vi "fetchChannelList.vi"(8 "error in":errorcluster, 10 "DAQ ID #":i32, 11 "Channels":string) -> (0 "error out":errorcluster, 2 "Channel Match?":bool, 3 "Read Channels":string)   [LabVIEW 2024]
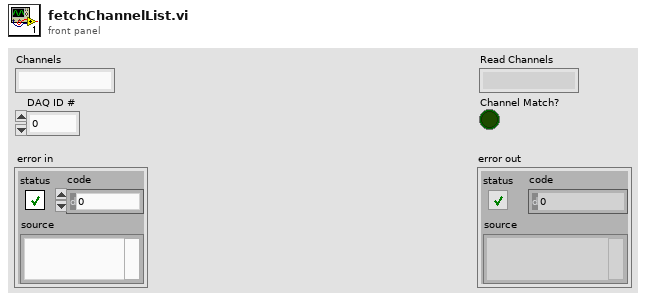
[diagram p1: front panel]
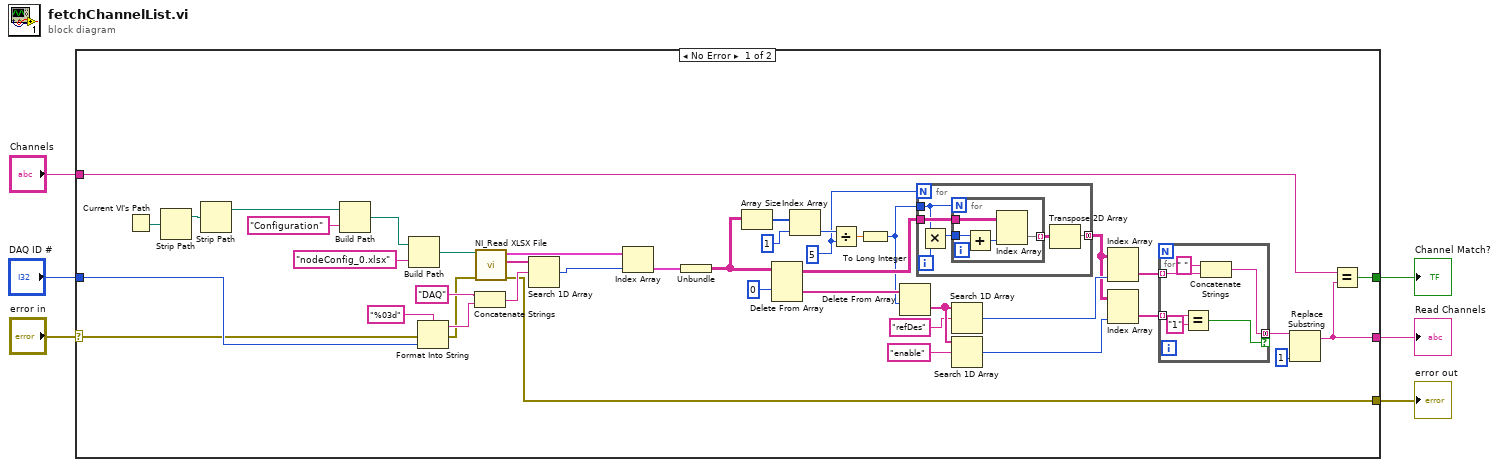
[diagram p0: block diagram]
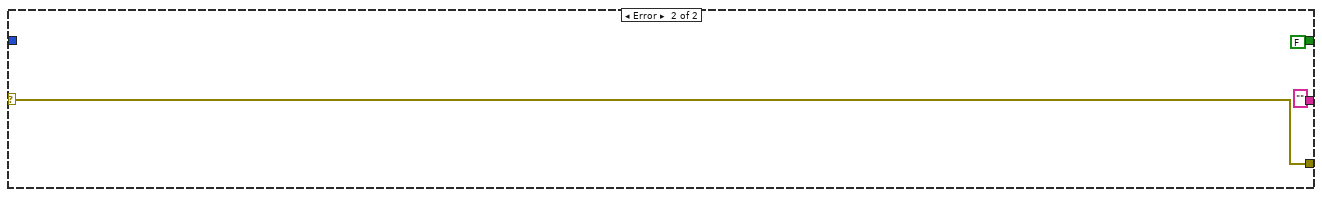
[diagram p2: hidden frame]
diagram:
  n1 = case shown="No Error" "error in" {
    selector: "error in" -> [w25 w66]
    tunnel: "DAQ ID #" -> [w32 _]
    tunnel: [w7 ""] -> w5
    tunnel: "Channels" -> [w15 _]
    tunnel: [w26 FALSE] -> w3
    tunnel: [w24 w66] -> w1
    frame No Error {
      w17 = 5 ("y")
      n2 = Current VI's Path() -> (path=w46:path)
      n3 = Strip Path(path=w46) -> (stripped path=w43:path)  [unwired: 1 out]
      n4 = Strip Path(path=w43) -> (stripped path=w42:path)  [unwired: 1 out]
      n5 = Build Path(base path=w42, name or relative path="Configuration") -> (appended path=w44:path)
      n6 = Build Path(base path=w44, name or relative path="nodeConfig_0.xlsx") -> (appended path=w47:path)
      n7 = Format Into String(format string="%03d", error in=w25, w32) -> (resulting string=w36:string, error out=w34:errorcluster)  [unwired: 1 in]
      n8 = Concatenate Strings("DAQ" ("string"), w36) -> (w38:string)
      n9 = call "NI_Read XLSX File.vi"("error in"=w34, "XLSX File"=w47) -> ("error out"=w24:errorcluster, "Sheet Names"=w39:string[], "Sheet Data"=w41:cluster{"Array":string[][]}[])  [unwired: 7 in]
      n10 = Search 1D Array(1D array=w39, element=w38) -> (index of element=w33:i32)  [unwired: 1 in]
      n11 = Index Array(array=w41, index=w33) -> (element=w40:cluster{"Array":string[][]})
      n12 = Unbundle(w40) -> ("Array"=w23:string[][])
      n13 = Array Size(array=w23) -> (size(s)=w31:i32[])
      n14 = Delete From Array(array=w23, index (row)=0) -> (deleted portion=w19:string[], array with subset deleted=w18:string[][])  [unwired: 2 in]
      n15 = Index Array(array=w31, index=1) -> (element=w29:i32)
      n16 = Divide(x=w29, y=w17) -> (x/y=w27:dbl)
      n17 = To Long Integer(number=w27) -> (32bit integer=w16:i32)
      n18 = Delete From Array(array=w19, length=w16) -> (deleted portion=w22:string[])  [unwired: 1 in, 1 out]
      n19 = for {
        N: w17 -> [_]
        tunnel: w18 -> [w60]
        tunnel: w16 -> [w58]
        tunnel: [w55] -> w13 mode=concatenating
        i -> [w59]
        n20 = Multiply(x=w58, y=w59) -> (x*y=w57:i32)
        n21 = for {
          N: w58 -> [_]
          tunnel: w60 -> [w65]
          tunnel: w57 -> [w63]
          tunnel: [w61] -> w56 mode=indexing
          i -> [w64]
          n22 = Add(x=w63, y=w64) -> (x+y=w62:i32)
          n23 = Index Array(array=w65, index (col)=w62) -> (element=w61:string[])  [unwired: 1 in]
        }
        n24 = Transpose 2D Array(2D array=w56) -> (transposed array=w55:string[][])
      }
      n25 = Search 1D Array(1D array=w22, element="refDes") -> (index of element=w14:i32)  [unwired: 1 in]
      n26 = Search 1D Array(1D array=w22, element="enable") -> (index of element=w12:i32)  [unwired: 1 in]
      n27 = Index Array(array=w13, index (col)=w14) -> (element=w11:string[])  [unwired: 1 in]
      n28 = Index Array(array=w13, index (col)=w12) -> (element=w10:string[])  [unwired: 1 in]
      n29 = for {
        tunnel: w11 -> [w54] mode=indexing
        tunnel: w10 -> [w51] mode=indexing
        tunnel: [w53] -> w9 mode=concatenating if=w49
        n30 = Equal?(x=w51, y="1") -> (x = y?=w49:bool)
        n31 = Concatenate Strings(" " ("string"), w54) -> (w53:string)
      }
      n32 = Replace Substring(2:1 ("length (len. of substring)"), 5:w9) -> (1:w7:string)  [unwired: 2 in, 1 out]
      n33 = Equal?(x=w15, y=w7) -> (x = y?=w26:bool)
    }
    frame Error {
    }
  }
  "error out" <- w1
  "Read Channels" <- w5
  "Channel Match?" <- w3
